vi "add.vi"() -> ()   [LabVIEW 2015]
panel:
  out "x+y":i32
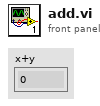
[diagram p1: front panel]
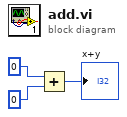
[diagram p0: block diagram]
diagram:
  n1 = Add(x=0, y=0) -> (x+y=→"x+y":i32)
